vi "PV ActiveLine - Are you there.vi"(0 "Referenz in":refnum<visa-resource-name>, 11 "Fehler (Eingang)":errorcluster) -> (4 "Referenz out":refnum<visa-resource-name>, 6 "Device Type":string, 8 "Serial Number":string, 10 "Article ID":string, 13 "Hardware Version":string, 14 "Firmware Version":string, 15 "Cluster (Ausgang)":errorcluster)   [LabVIEW 2013, in "PV ActiveLine.lvlib"]
doc: "AYT - System Information\n\nReceive: a,b,c,d,e\n\na - Type of the unit, e.g. TPG362\nb - Model No. of the unit, e.g. PTG28290\nc - Serial No. of the unit, e.g. 44990000\nd - Firmware version of the unit, e.g.. 010100\ne - Hardware version of the unit, e.g. 010100"
uses:
  C:/Program Files (x86)/National Instruments/LabVIEW 2013/PV ActiveLine/PV ActiveLine.lvlib
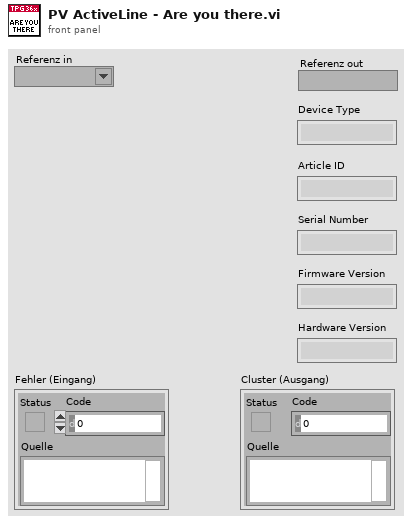
[diagram p1: front panel]
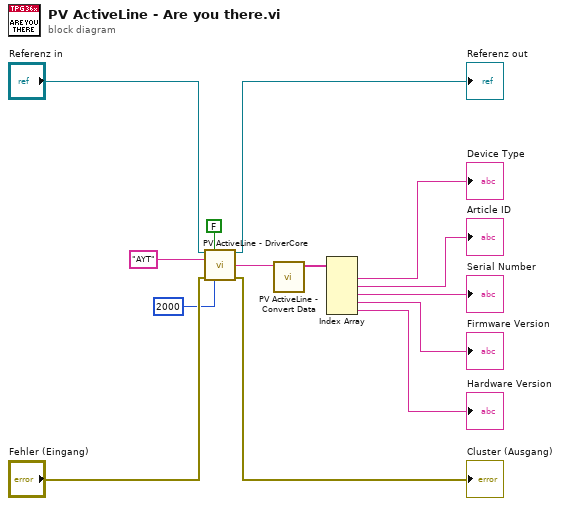
[diagram p0: block diagram]
diagram:
  n1 = call "PV ActiveLine - DriverCore.vi"("Referenz in"="Referenz in", "Write/Read"=FALSE, "Command"="AYT", "Fehler (Eingang)"="Fehler (Eingang)", "Timeout [ms]"=u32 2000) -> ("Referenz out"=→"Referenz out":refnum<visa-resource-name>, "String Out"=w8:string, "Cluster (Ausgang)"=→"Cluster (Ausgang)":errorcluster)  [unwired: 8 in]
  n2 = call "PV ActiveLine - Convert Data.vi"("String in"=w8) -> ("String out"=w7:string[])  [unwired: 7 in, 3 out]
  n3 = Index Array(array=w7) -> (element #1=→"Device Type":string, element #2=→"Article ID":string, element #3=→"Serial Number":string, element #4=→"Firmware Version":string, element #5=→"Hardware Version":string)  [unwired: 5 in]
